vi "SCE_color_palette.vi"(9 "color index":u8) -> (1 "selected color":u32(colorbox), 2 "color palette":u32[](array[colorbox])=[0, 16777215, 8912896, 11206638, 13386956, 52309, 170, 15658615, 14518357, 6702080, 16742263, 3355443, 7829367, 11206502, 35071, 12303291])   [LabVIEW 2018]
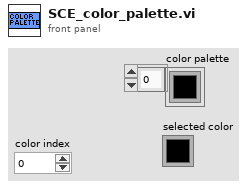
[diagram p1: front panel]
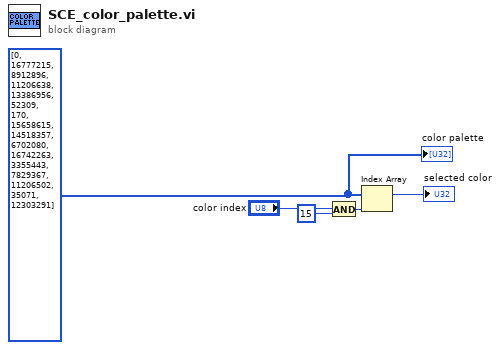
[diagram p0: block diagram]
diagram:
  w3 = u32[] [0, 16777215, 8912896, 11206638, 13386956, 52309, 170, 15658615, 14518357, 6702080, 16742263, 3355443, 7829367, 11206502, 35071, 12303291] ("color table")
  n1 = And(x="color index", y=u8 15) -> (x .and. y?=w4:u8)
  n2 = Index Array(array=w3, index=w4) -> (element=→"selected color":u32)
  "color palette" <- w3
